vi "Inerpol.vi"(9 "ArrayChastot":dbl[][](array[numeric]), 10 "All GLUBIN":dbl[](array[numeric]), 11 "all rows":string[][](array[string])=[["", "50000", "100000", "200000"], ["100", "0", "0", "0"], ["75.3", "-11.3", "-21.7", "-46.55"], ["55.3", "-19.9", "-30.2", "-69.65"], ["35.3", "-30", "-47.2", "-109.2"], ["", "", "", ""], ["", "", "", ""], ["", "", "", ""]]) -> (3 "appended array":string[][](array[string]))   [LabVIEW 2017]
uses:
  <vilib>/Analysis/NI_AALPro.lvlib
panel:
  out "intercept":dbl
  out "0Glubina":dbl[](array[numeric])
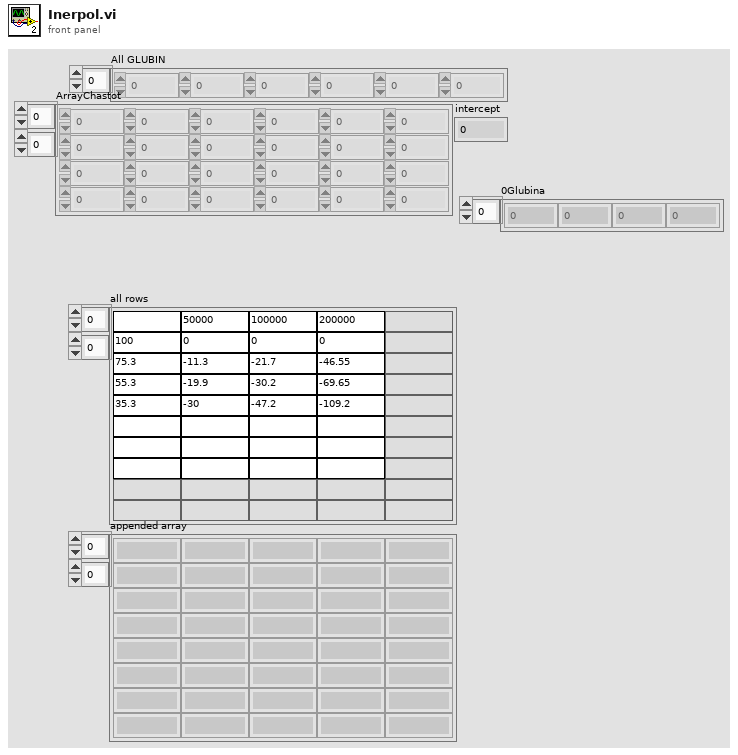
[diagram p1: front panel]
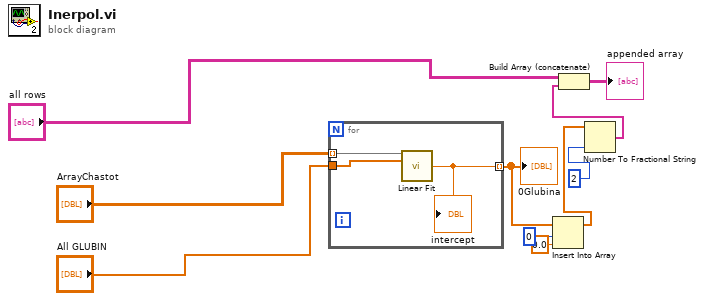
[diagram p0: block diagram]
diagram:
  n1 = for {
    tunnel: "ArrayChastot" -> [w13] mode=indexing
    tunnel: "All GLUBIN" -> [w12]
    tunnel: [w11] -> w4 mode=indexing
    n2 = call <vilib>:"Linear Fit.vi"("Y"=w13, "X"=w12) -> ("intercept"=w11:dbl)  [unwired: 9 in, 4 out]
    "intercept" <- w11
  }
  "0Glubina" <- w4
  n3 = Insert Into Array(array=w4, index=0, new element=0.0 ("new element/subarray")) -> (w1:dbl[])
  n4 = Number To Fractional String(number=w1, precision (6)=i16 2) -> (F-format string=w7:string[])  [unwired: 2 in]
  n5 = Build Array (concatenate)("all rows", w7) -> (→"appended array":string[][])
